vi "read_analog_worker_loop.vi"(7 "data_queues":cluster{"AnalogReadData":refnum<queue>}, 8 "error in (no error)":errorcluster, 9 "data_notifiers":T1, 10 "Notifiers":T3, 11 "Message Queues":T2) -> (0 "error out":errorcluster)   [LabVIEW 2017]
uses:
  support/Notifiers/Notifiers.ctl
  support/Message Queue/All Message Queues.ctl
  support/Message Queue/Message Cluster.ctl
  support/data_notifiers/data_Notifiers.ctl
  measurement_result/MeasurementResult.lvclass
  support/measurement_state.ctl
  measurement/Measurement.lvclass
  sim_hardware/SimHardware.lvclass
  C:/Users/mngoc/workspace/LDC/Zylinderkopfpruefstand/code/server/hardware/Hardware.lvclass
  hardware/hardware_type.ctl
  support/Message Queue/Enqueue Message (Single).vi
  <vilib>/Utility/error.llb/Error Cluster From Error Code.vi
  <vilib>/ErrorRing/Error Ring.xnode
  support/Message Queue/Message Queue.lvlib
  hardware/Hardware.lvclass
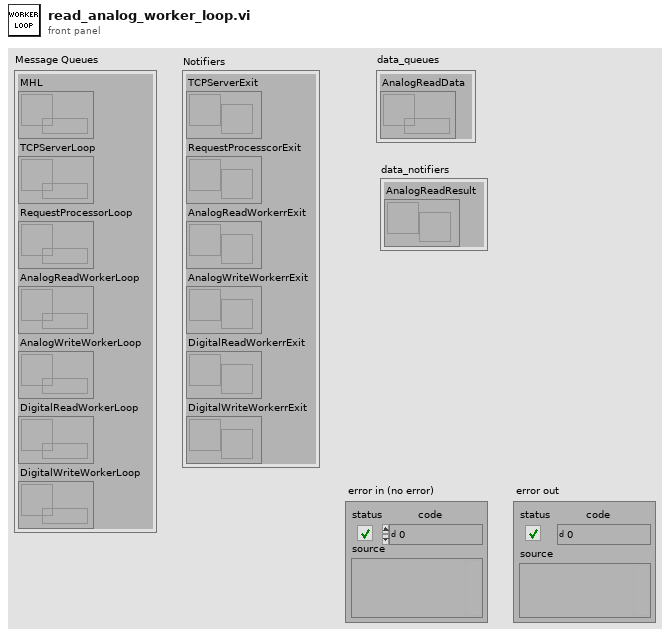
[diagram p1: front panel]
types:
  T1 = typedef "data_Notifiers.ctl" = cluster{"AnalogReadResult":refnum<notifier>}
  T2 = typedef "Message Queue.lvlib/All Message Queues.ctl" = cluster{"MHL":refnum<queue>, "TCPServerLoop":refnum<queue>, "RequestProcessorLoop":refnum<queue>, "AnalogReadWorkerLoop":refnum<queue>, "AnalogWriteWorkerLoop":refnum<queue>, "DigitalReadWorkerLoop":refnum<queue>, "DigitalWriteWorkerLoop":refnum<queue>}
  T3 = typedef "Notifiers.ctl" = cluster{"TCPServerExit":refnum<notifier>, "RequestProcesscorExit":refnum<notifier>, "AnalogReadWorkerrExit":refnum<notifier>, "AnalogWriteWorkerrExit":refnum<notifier>, "DigitalReadWorkerrExit":refnum<notifier>, "DigitalWriteWorkerrExit":refnum<notifier>}
  T4 = typedef "measurement_state.ctl" = enum16{"idle", "running"}
  T5 = typedef "Hardware.lvclass/hardware_type.ctl" = enum16{"Sim_Hardware", "AI_Ni_Hardware", "AO_Ni_Hardware", "DI_Ni_Hardware", "DO_Ni_Hardware"}
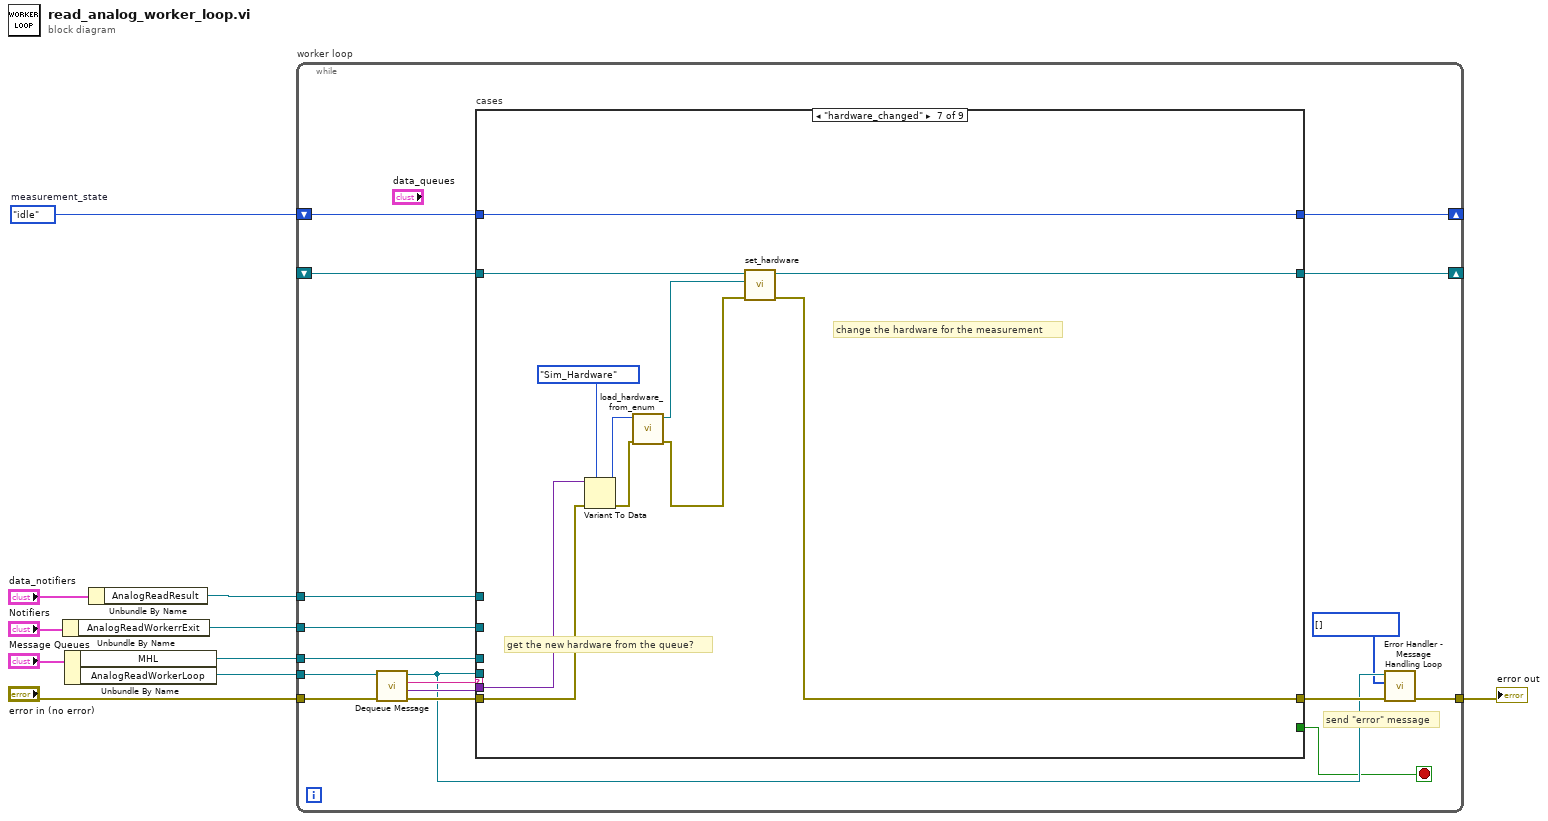
[diagram p0: block diagram]
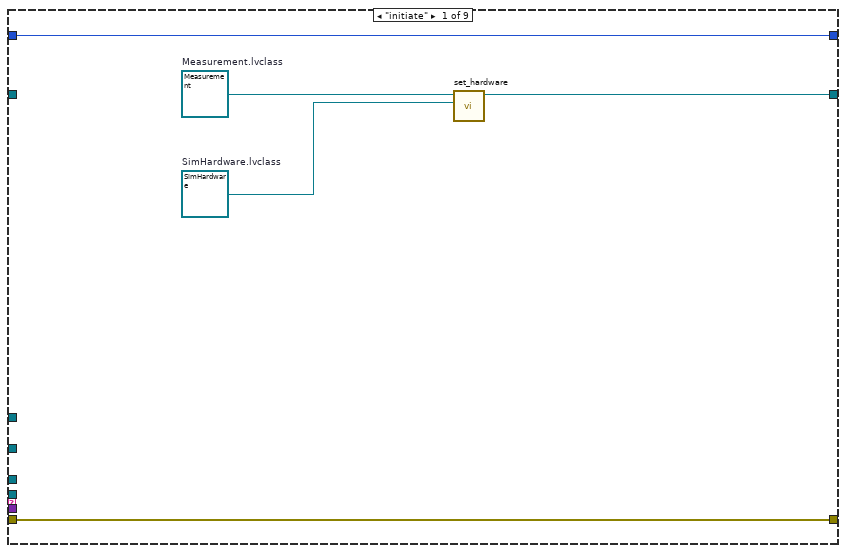
[diagram p2: hidden frame]
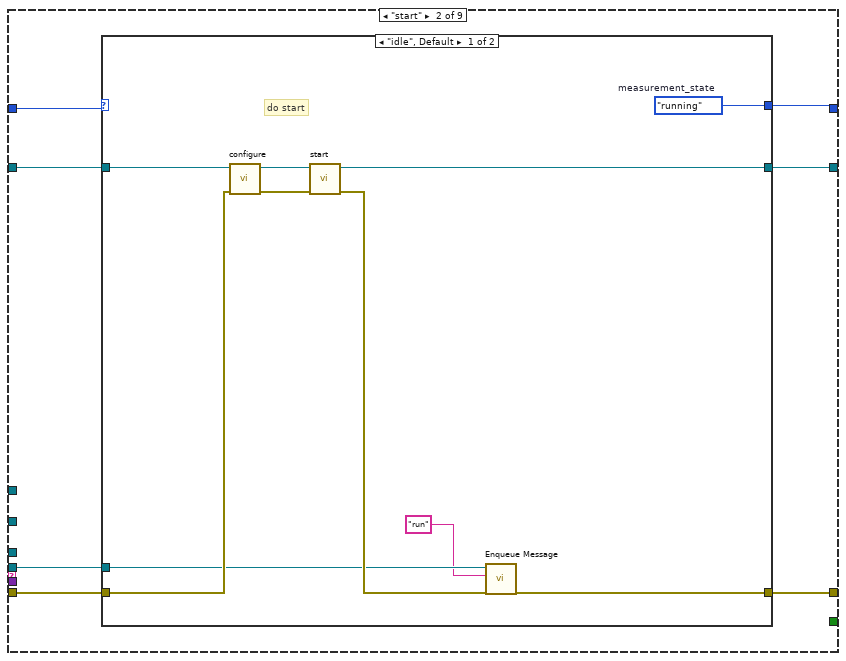
[diagram p3: hidden frame]
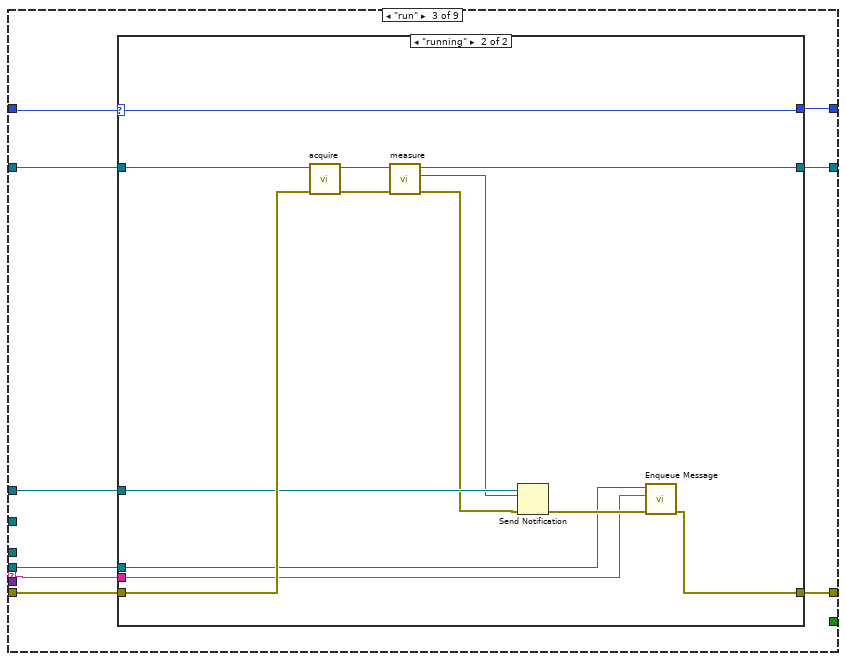
[diagram p5: hidden frame]
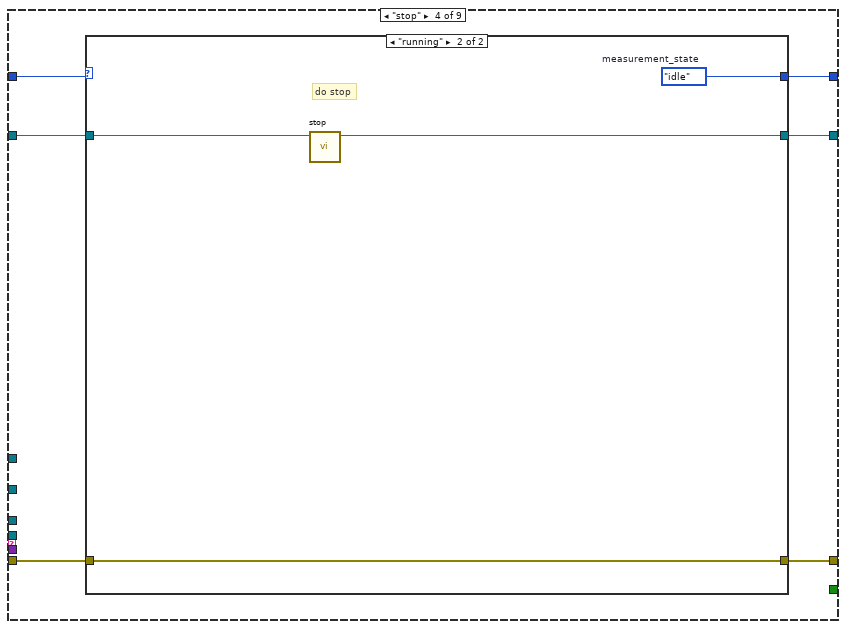
[diagram p7: hidden frame]
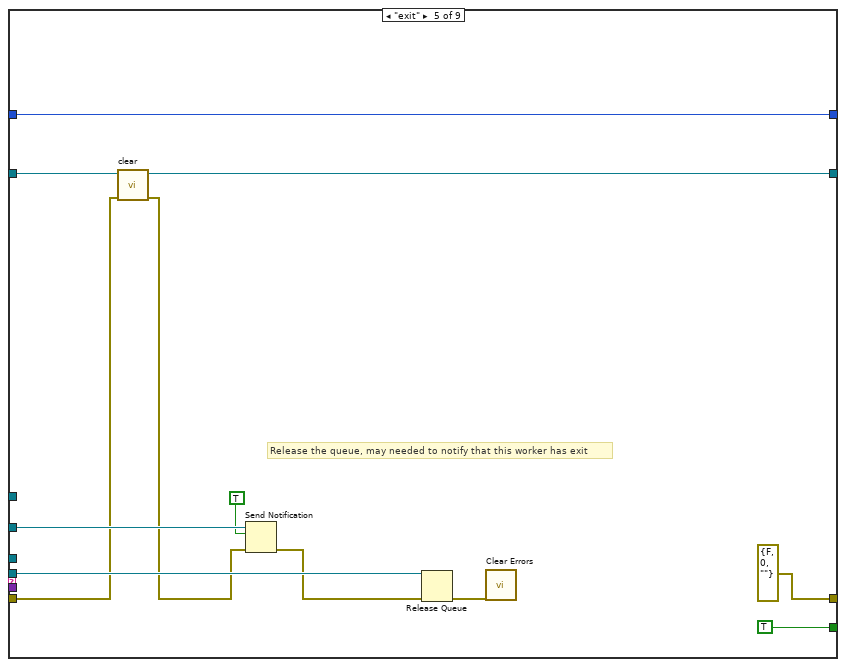
[diagram p9: hidden frame]
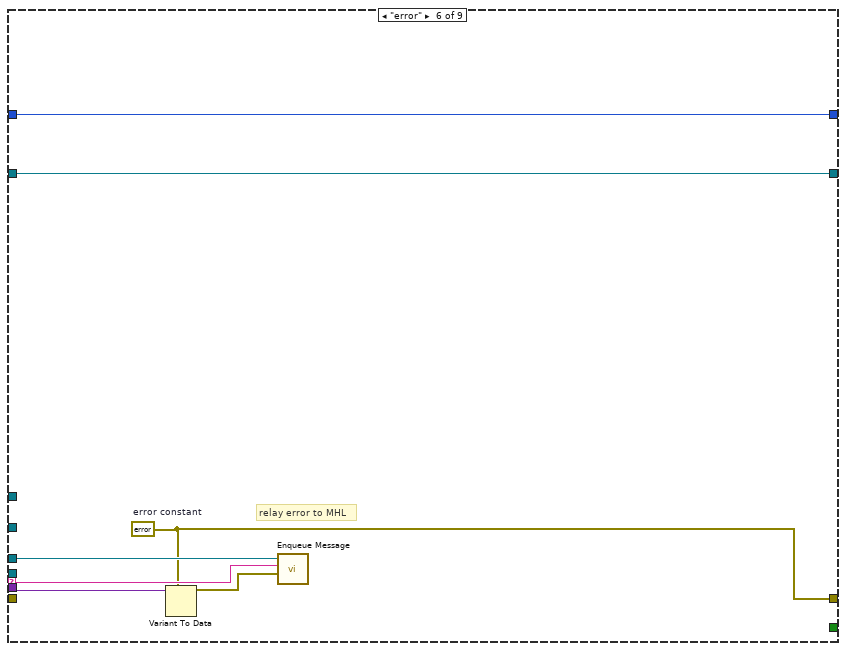
[diagram p10: hidden frame]
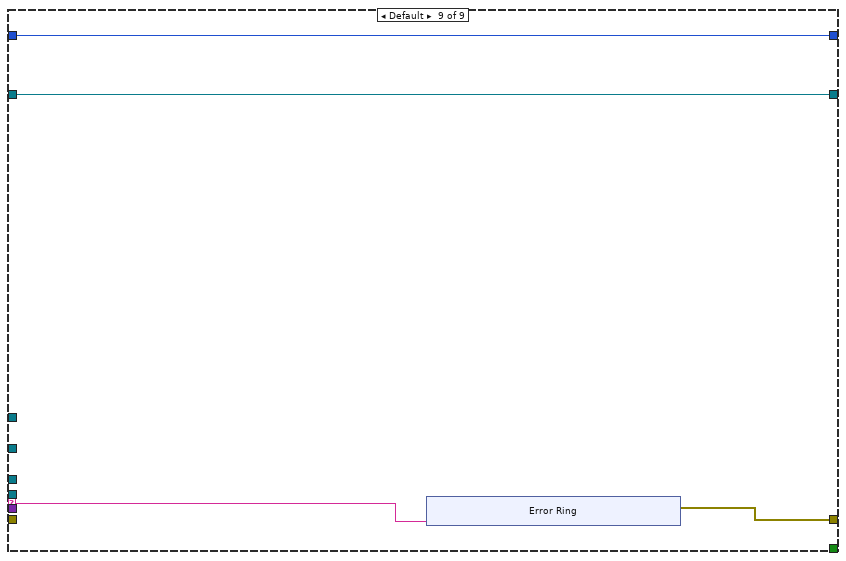
[diagram p12: hidden frame]
diagram:
  w3 = measurement_state."idle"  # measurement_state
  n1 = Unbundle By Name("Notifiers") -> ("AnalogReadWorkerrExit"=w4:refnum<notifier>)
  n2 = Unbundle By Name("Message Queues") -> ("MHL"=w6:refnum<queue>, "AnalogReadWorkerLoop"=w7:refnum<queue>)
  n3 = Unbundle By Name("data_notifiers") -> ("AnalogReadResult"=w1:refnum<notifier>)
  n4 = while "worker loop" {
    tunnel: "error in (no error)" -> [w27]
    tunnel: [w22] -> w9
    tunnel: w7 -> [w18]
    tunnel: w6 -> [w17]
    tunnel: w4 -> [w16]
    shift-right: [w14] -> _
    shift-left: w3 -> [w15]
    shift-right: [w13] -> _
    shift-left: _ -> [w12]
    tunnel: w1 -> [w11]
    stop <- w19 stop-if-true
    # "send \"error\" message"
    n5 = call "Dequeue Message.vi"("error in (no error)"=w27, "Message Queue"=w18) -> ("error out"=w26:errorcluster, "Message Data"=w24:variant, "Message"=w25:string, "dup Message Queue"=w21:refnum<queue>)  [unwired: 6 in]
    n6 = case "cases" shown="\"hardware_changed\"" w25 {
      selector: w25 -> [_ _ w53 _ _ w109 _ _ w127]
      tunnel: w26 -> [w32 w39 w59 w83 w93 _ w114 w123 _]
      tunnel: [w32 w38 w58 w82 errorcluster {"status"=FALSE, "code"=0, "source"=""} ("error constant") w105 w117 w123 w126] -> w23
      tunnel: w24 -> [_ _ _ _ _ w108 w115 _ _]
      tunnel: w21 -> [_ w33 w54 _ w100 _ _ _ _]
      tunnel: [_ _ _ _ TRUE _ _ _ _] -> w19
      tunnel: w17 -> [_ _ _ _ _ w106 _ _ _]
      tunnel: w16 -> [_ _ _ _ w99 _ _ _ _]
      tunnel: w15 -> [w31 w37 w61 w81 w96 w104 w120 w122 w125]
      tunnel: [w31 w36 w60 w80 w96 w104 w120 w122 w125] -> w14
      tunnel: [w29 w34 w56 w78 w94 w103 w118 w121 w124] -> w13
      tunnel: w12 -> [_ w35 w57 w79 w95 w103 w119 w121 w124]
      tunnel: w11 -> [_ _ w55 _ _ _ _ _ _]
      frame "initiate" {
        w28 = refnum<class "SimHardware.lvclass"> refnum  # SimHardware.lvclass
        w30 = refnum<class "Measurement.lvclass"> refnum  # Measurement.lvclass
        n7 = call "set_hardware.vi"("new_hardware"=w28, "Measurement in"=w30) -> ("Measurement out"=w29:refnum<class "Measurement.lvclass">)  [unwired: 8 in, 1 out]
      }
      frame "start" {
        n8 = case shown="\"idle\", Default" w37 {
          selector: w37 -> [_ w51]
          tunnel: w39 -> [w45 w52]
          tunnel: [w42 w52] -> w38
          tunnel: [w49 w51] -> w36
          tunnel: w35 -> [w47 w50]
          tunnel: [w48 w50] -> w34
          tunnel: w33 -> [w41 _]
          frame "idle", Default {
            w49 = measurement_state."running"  # measurement_state
            # "do start"
            n9 = call-dynamic "configure.vi"("error in (no error)"=w45, "Measurement in"=w47) -> ("error out"=w44:errorcluster, "Measurement out"=w46:refnum<class "Measurement.lvclass">)  [unwired: 8 in]
            n10 = call-dynamic "start.vi"("error in (no error)"=w44, "Measurement in"=w46) -> ("error out"=w43:errorcluster, "Measurement out"=w48:refnum<class "Measurement.lvclass">)  [unwired: 8 in]
            n11 = call-poly "Enqueue Message.vi"("error in (no error)"=w43, "Message"="run", "Message Queue"=w41) -> ("error out"=w42:errorcluster)  [unwired: 7 in, 1 out]
          }
          frame "running" {
            # "already running -> do nothing"
          }
        }
      }
      frame "run" {
        n12 = case shown="\"running\"" w61 {
          selector: w61 -> [w64 w77]
          tunnel: [w64 w77] -> w60
          tunnel: w59 -> [w63 w75]
          tunnel: [w63 w65] -> w58
          tunnel: w57 -> [w62 w76]
          tunnel: [w62 w73] -> w56
          tunnel: w55 -> [_ w71]
          tunnel: w54 -> [_ w67]
          tunnel: w53 -> [_ w66]
          frame "idle", Default {
            # "do nothing"
          }
          frame "running" {
            n13 = call-dynamic "acquire.vi"("error in (no error)"=w75, "Measurement in"=w76) -> ("error out"=w72:errorcluster, "Measurement out"=w74:refnum<class "Measurement.lvclass">)  [unwired: 8 in]
            n14 = call-dynamic "measure.vi"("error in (no error)"=w72, "Measurement in"=w74) -> ("error out"=w69:errorcluster, "result"=w70:refnum<class "MeasurementResult.lvclass">, "Measurement out"=w73:refnum<class "Measurement.lvclass">)  [unwired: 7 in]
            n15 = Send Notification(notification=w70, notifier=w71, error in (no error)=w69) -> (error out=w68:errorcluster)  [unwired: 1 out]
            n16 = call-poly "Enqueue Message.vi"("error in (no error)"=w68, "Message"=w66, "Message Queue"=w67) -> ("error out"=w65:errorcluster)  [unwired: 7 in, 1 out]
          }
        }
      }
      frame "stop" {
        n17 = case shown="\"running\"" w81 {
          selector: w81 -> [w85 _]
          tunnel: w83 -> [w86 w90]
          tunnel: [w86 w90] -> w82
          tunnel: [w85 w89] -> w80
          tunnel: w79 -> [w84 w88]
          tunnel: [w84 w87] -> w78
          frame "idle", Default {
            # "do nothing"
          }
          frame "running" {
            w89 = measurement_state."idle"  # measurement_state
            # "do stop"
            n18 = call-dynamic "stop.vi"("Measurement in"=w88) -> ("Measurement out"=w87:refnum<class "Measurement.lvclass">)  [unwired: 9 in, 1 out]
          }
        }
      }
      frame "exit" {
        # "Release the queue, may needed to notify that this worker has exit"
        n19 = call-dynamic "clear.vi"("error in (no error)"=w93, "Measurement in"=w95) -> ("error out"=w92:errorcluster, "Measurement out"=w94:refnum<class "Measurement.lvclass">)  [unwired: 8 in]
        n20 = Send Notification(notification=TRUE, notifier=w99, error in (no error)=w92) -> (error out=w98:errorcluster)  [unwired: 1 out]
        n21 = Release Queue(queue=w100, error in (no error)=w98) -> (error out=w91:errorcluster)  [unwired: 1 in, 2 out]
        n22 = call <vilib>:"Clear Errors.vi"("error in (no error)"=w91) -> ()  [unwired: 5 in, 2 out]
      }
      frame "error" {
        w105 = errorcluster {"status"=FALSE, "code"=0, "source"=""}  # error constant
        # "relay error to MHL"
        n23 = Variant To Data(type=w105, Variant=w108) -> (data=w107:errorcluster)  [unwired: 1 in, 1 out]
        n24 = call-poly "Enqueue Message.vi"("Message Data"=w107, "Message"=w109, "Message Queue"=w106) -> ()  [unwired: 7 in, 2 out]
      }
      frame "hardware_changed" {
        # "get the new hardware from the queue?"
        # "change the hardware for the measurement"
        n25 = Variant To Data(error in=w114, type=hardware_type."Sim_Hardware" ("hardware type"), Variant=w115) -> (data=w113:T5, error out=w111:errorcluster)
        n26 = call "load_hardware_from_enum.vi"("error in (no error)"=w111, "hardware type"=w113) -> ("error out"=w110:errorcluster, "Hardware out"=w112:refnum<class "Hardware.lvclass">)  [unwired: 8 in]
        n27 = call "set_hardware.vi"("error in (no error)"=w110, "new_hardware"=w112, "Measurement in"=w119) -> ("error out"=w117:errorcluster, "Measurement out"=w118:refnum<class "Measurement.lvclass">)  [unwired: 7 in]
      }
      frame "duplicate_me" {
      }
      frame Default {
        n28 = xnode "Error Ring"("parameter 0"=w127) -> ("error out"=w126:errorcluster)
      }
    }
    n29 = call "Error Handler - Message Handling Loop.vi"("error in (no error)"=w23, "Ignore Errors (Runtime)"=i32[] [], "Message Queue"=w21) -> ("dup error in"=w22:errorcluster)  [unwired: 7 in, 1 out]
  }
  "error out" <- w9
